vi "Plot Editor_Remove out-of-bound Plot Values.vi"(6 "Control Refnums":refnum<vi>[](array[refnum]), 7 "XYGraph in":refnum<vi>, 8 "error in (no error)":errorcluster, 11 "Plot Editor Internal Data":T1) -> (0 "error out":errorcluster, 2 "Message":string, 3 "Plot Editor Internal Data out":T1)   [LabVIEW 2021, in "Plot Editor.lvlib"]
uses:
  Plot Editor.lvlib
  Plot Editor Internal Variables.ctl
  XY Graph/XY Graph Plot Properties.ctl
  XY Graph/XY Graph Add-Ons.lvlib
panel:
  in  "Array":refnum<vi>
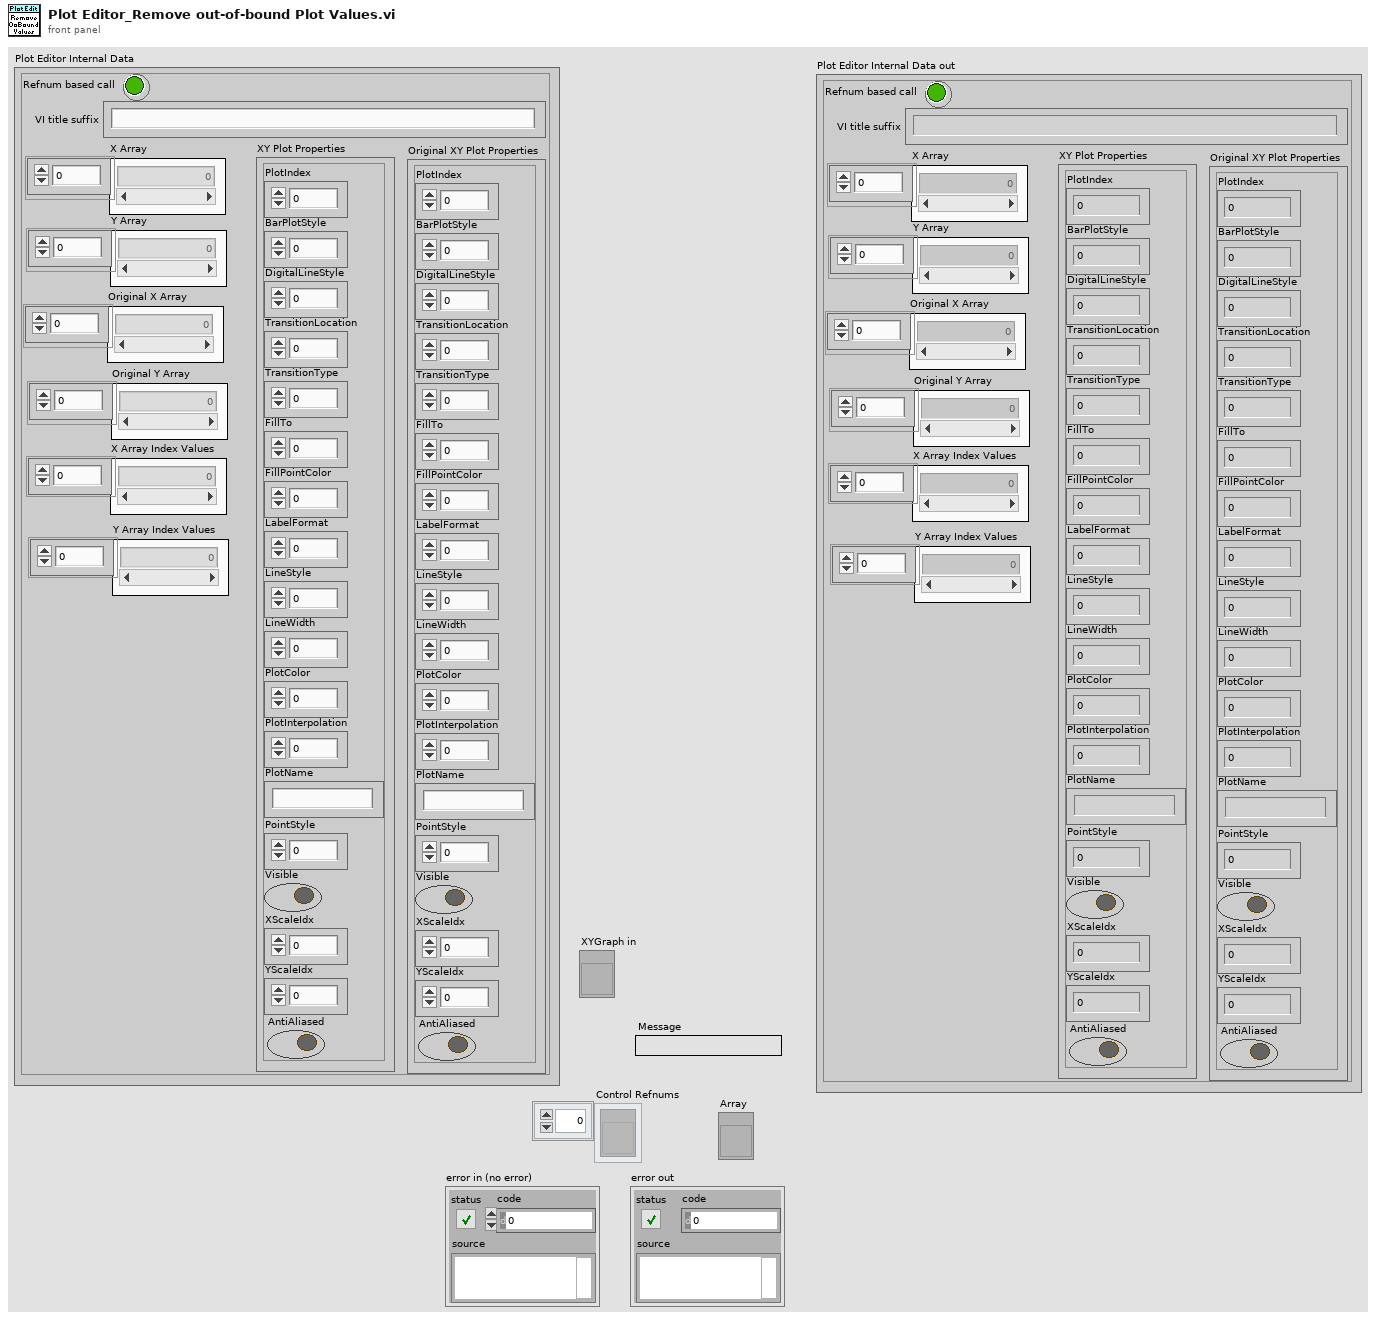
[diagram p1: front panel]
types:
  T1 = typedef "Plot Editor.lvlib/Plot Editor Internal Variables.ctl" = cluster{"X Array":dbl[], "Y Array":dbl[], "XY Plot Properties":T2, "X Array Index Values":u32[], "Y Array Index Values":u32[], "Original XY Plot Properties":T2, "Original X Array":dbl[], "Original Y Array":dbl[], "VI title suffix":string, "Refnum based call":bool}
  T2 = typedef "XY Graph Add-Ons.lvlib/XY Graph Plot Properties.ctl" = cluster{"PlotIndex":i32, "BarPlotStyle":u8, "DigitalLineStyle":u8, "TransitionLocation":u8, "TransitionType":u8, "FillTo":i16, "FillPointColor":u32, "LabelFormat":u8, "LineStyle":u8, "LineWidth":u8, "PlotColor":u32, "PlotInterpolation":u8, "PlotName":string, "PointStyle":u8, "Visible":bool, "XScaleIdx":u32, "YScaleIdx":u32, "AntiAliased":bool}
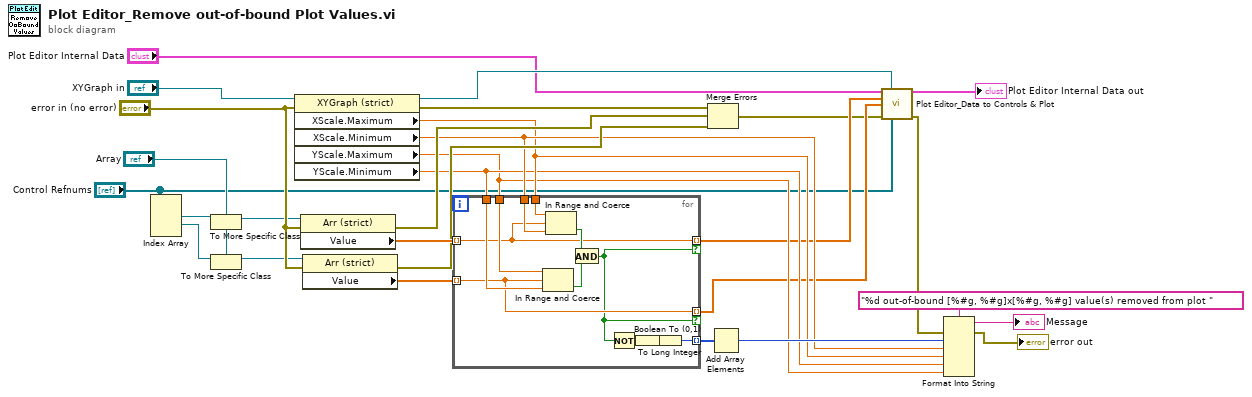
[diagram p0: block diagram]
diagram:
  n1 = Index Array(array="Control Refnums") -> (element #1=w14:refnum<vi>, element #2=w12:refnum<vi>)  [unwired: 3 in, 1 out]
  n2 = To More Specific Class(target class="Array", reference=w14) -> (specific class reference=w13:refnum<vi>)  [unwired: 1 in, 1 out]
  n3 = To More Specific Class(target class="Array", reference=w12) -> (specific class reference=w11:refnum<vi>)  [unwired: 1 in, 1 out]
  n4 = property class="XYGraph (strict)"(reference="XYGraph in", error in="error in (no error)") -> (reference out=w5:refnum<vi>, error out=w25:errorcluster, "XScale.Maximum"=w19:dbl, "XScale.Minimum"=w20:dbl, "YScale.Maximum"=w17:dbl, "YScale.Minimum"=w18:dbl)
  n5 = property class="Arr (strict)"(reference=w13, error in="error in (no error)") -> (error out=w24:errorcluster, "Value"=w28:dbl[])  [unwired: 1 out]
  n6 = property class="Arr (strict)"(reference=w11, error in="error in (no error)") -> (error out=w23:errorcluster, "Value"=w27:dbl[])  [unwired: 1 out]
  n7 = for {
    tunnel: w28 -> [w35] mode=indexing
    tunnel: w27 -> [w34] mode=indexing
    tunnel: w19 -> [w41]
    tunnel: w20 -> [w40]
    tunnel: w17 -> [w39]
    tunnel: w18 -> [w38]
    tunnel: [w35] -> w9 mode=indexing if=w33
    tunnel: [w34] -> w8 mode=indexing if=w33
    tunnel: [w31] -> w22 mode=indexing
    n8 = In Range and Coerce(upper limit=w39, x=w34, lower limit=w38) -> (In Range?=w36:bool)  [unwired: 1 out]
    n9 = In Range and Coerce(upper limit=w41, x=w35, lower limit=w40) -> (In Range?=w37:bool)  [unwired: 1 out]
    n10 = And(x=w37, y=w36) -> (x .and. y?=w33:bool)
    n11 = Not(x=w33) -> (.not. x?=w30:bool)
    n12 = Boolean To (0,1)(Boolean=w30) -> (0, 1=w32:i16)
    n13 = To Long Integer(number=w32) -> (32bit integer=w31:i32)
  }
  n14 = Merge Errors(w25, w24, w23) -> (w7:errorcluster)
  n15 = Add Array Elements(numeric array=w22) -> (sum=w21:i32)
  n16 = call "Plot Editor_Data to Controls & Plot.vi"("Plot Editor Internal Data"="Plot Editor Internal Data", "XYGraph in"=w5, "X Array"=w9, "Y Array"=w8, "error in (no error)"=w7, "Control Refnums"="Control Refnums") -> ("Plot Editor Internal Data"=→"Plot Editor Internal Data out":T1, "error out"=w2:errorcluster)  [unwired: 8 in]
  n17 = Format Into String(format string="%d out-of-bound [%#g, %#g]x[%#g, %#g] value(s) removed from plot ", error in=w2, w21, w20, w19, w18, w17) -> (resulting string=→"Message":string, error out=→"error out":errorcluster)  [unwired: 1 in]
